vi "getCurrentMission.vi"(8 "error in (no error)":errorcluster, 10 "Current Mission In":refnum<class "GenericMission.lvclass">, 11 "MissionQueue in":refnum<class "MissionQueue.lvclass">) -> (0 "error out":errorcluster, 2 "Mission Out":refnum<class "GenericMission.lvclass">, 3 "MissionQueue out":refnum<class "MissionQueue.lvclass">)   [LabVIEW 2011, in "MissionQueue.lvclass"]
doc: "Remove and return the first element from the queue. If the queue is not empty, the \"valid?\" flag will be True."
uses:
  MissionQueue.lvclass
  Missions/GenericMission/GenericMission.lvclass
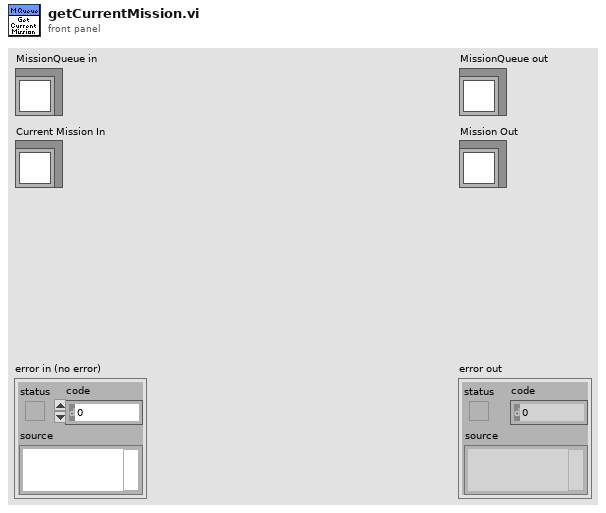
[diagram p1: front panel]
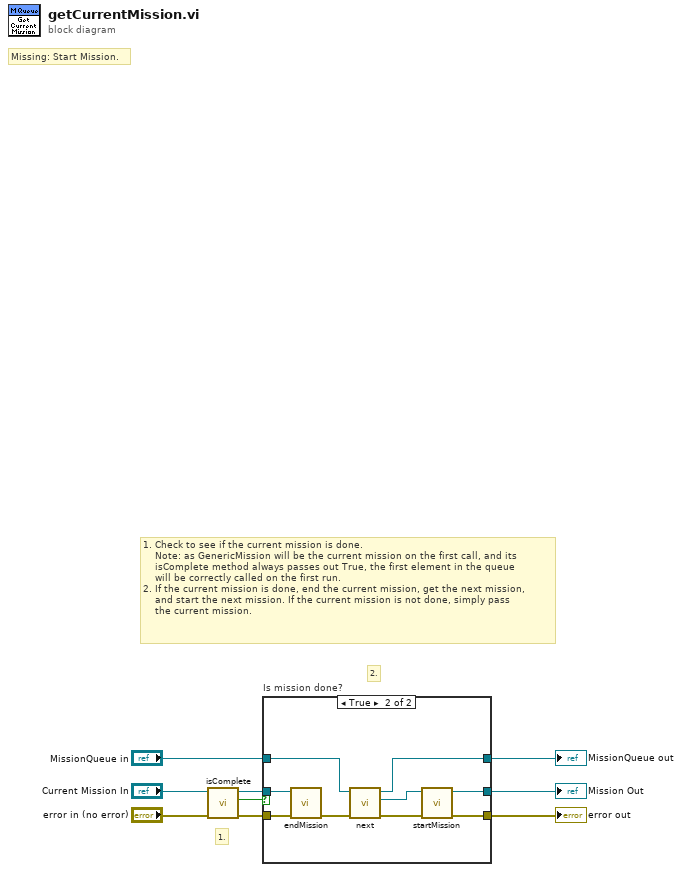
[diagram p0: block diagram]
diagram:
  # "2."
  # "1."
  # "1. Check to see if the current mission is done.\n    Note: as GenericMission will be the current mission on the first call, and its\n    isComplete method always passes out True, the first element in the queue\n    will be correctly called on the first run.\n2. If the current mission is done, end the current mission, get the next mission,\n    and start the next mission. If the current mission is not done, simply pass\n    the current mission."
  # "Missing: Start Mission."
  n1 = call-dynamic "isComplete.vi"("error in (no error)"="error in (no error)", "Mission in"="Current Mission In") -> ("error out"=w7:errorcluster, "Mission Complete?"=w9:bool, "Mission out"=w8:refnum<class "GenericMission.lvclass">)  [unwired: 7 in]
  n2 = case "Is mission done?" shown="True" w9 {
    tunnel: w8 -> [w12 w21]
    tunnel: w7 -> [w10 w20]
    tunnel: [w12 w15] -> w4
    tunnel: "MissionQueue in" -> [w11 w18]
    tunnel: [w10 w14] -> w3
    tunnel: [w11 w13] -> w2
    frame False {
    }
    frame True {
      n3 = call-dynamic "endMission.vi"("error in (no error)"=w20, "GenericMission in"=w21) -> ("error out"=w19:errorcluster)  [unwired: 8 in, 1 out]
      n4 = call "next.vi"("error in (no error)"=w19, "MissionQueue in"=w18) -> ("error out"=w16:errorcluster, "GenericMission.lvclass"=w17:refnum<class "GenericMission.lvclass">, "MissionQueue out"=w13:refnum<class "MissionQueue.lvclass">)  [unwired: 6 in, 1 out]
      n5 = call-dynamic "startMission.vi"("error in (no error)"=w16, "GenericMission in"=w17) -> ("error out"=w14:errorcluster, "GenericMission out"=w15:refnum<class "GenericMission.lvclass">)  [unwired: 8 in]
    }
  }
  "error out" <- w3
  "MissionQueue out" <- w2
  "Mission Out" <- w4
